vi "TRIG_CHAN_AUX_INT.vi"(0 "VISA IN":refnum<visa-resource-name>, 1 "Aux":i32, 2 "Interval":string(combo)="SWE", 5 "error in":errorcluster, 7 "Channel":i32) -> (14 "VISA Out":refnum<visa-resource-name>, 19 "error out":errorcluster)   [LabVIEW 2018, in "PNA-X.lvlib"]
doc: "TRIGger:CHANnel<ch>:AUX<n>:INTerval <char> \n1889\n\n(Read-Write) Specifies how often a trigger output signal is sent. \nParameters \n<ch> Any existing channel number. If unspecified, value is set to 1. \n<n> Rear panel connector used to send or receive signals. \nPNA-X - choose from 1 (AUX TRIG 1) or 2 (AUX TRIG 2) \nAll other models: choose 1. (BNC Trig I/O \nIf unspecified, value is set to 1. \n<char> Choose from: \nPOINt Trigger signal is sent every data point. (effectively the same as Point \nsweep) \nSWEep Trigger signal is sent once every sweep. \nExamples TRIG:CHAN:AUX:INT POI \ntrigger:channel2:aux2:interval sweep \nQuery Syntax TRIGger:CHANnel<ch>:AUX<n>:INTerval? \nReturn Type Character \nDefault SWEep"
uses:
  PNA-X.lvlib
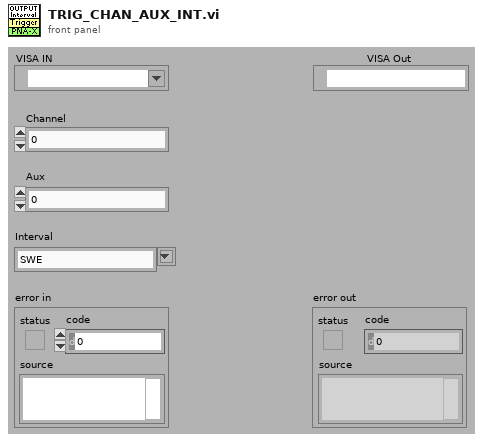
[diagram p1: front panel]
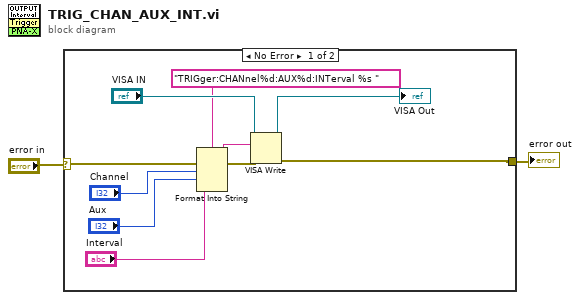
[diagram p0: block diagram]
diagram:
  n1 = case shown="No Error" "error in" {
    selector: "error in" -> [w12 w13]
    tunnel: [w7 w13] -> w1
    frame No Error {
      n2 = Format Into String(format string="TRIGger:CHANnel%d:AUX%d:INTerval %s " ("Cmdline"), error in=w12, "Channel", "Aux", "Interval") -> (resulting string=w10:string, error out=w11:errorcluster)  [unwired: 1 in]
      n3 = VISA Write(VISA resource name="VISA IN", write buffer=w10, error in (no error)=w11) -> (VISA resource name out=→"VISA Out":refnum<visa-resource-name>, error out=w7:errorcluster)  [unwired: 1 out]
    }
    frame Error {
    }
  }
  "error out" <- w1
